vi "CLD 11 Producer consumer events solution.vi"() -> ()   [LabVIEW 2018]
doc: "CLD 11 exercise.\n\nThis VI uses the producer consumer architecture with an event structure. Since there was only one data value (time target) to be used, monitoring changes for the time target control is done with polling instead of the event structure."
uses:
  CLD 11 producer consumer enum.ctl
  CLD 11 CSV file data structure.ctl
  CLD 11 Producer Consumer Data Structure.ctl
  CLD 11 CSV file enum.ctl
panel:
  out "Current Time target":dbl
  out "Elapsed Time (s)":dbl
  out "Step 3":bool
  out "Step 2":bool
  out "Step 1":bool
  out "Time Has Elapsed":bool
  in  "Auto Reset":bool=TRUE
  in  "Reset Button":bool
  in  "Stop VI":bool
  in  "Time Target (s)":dbl
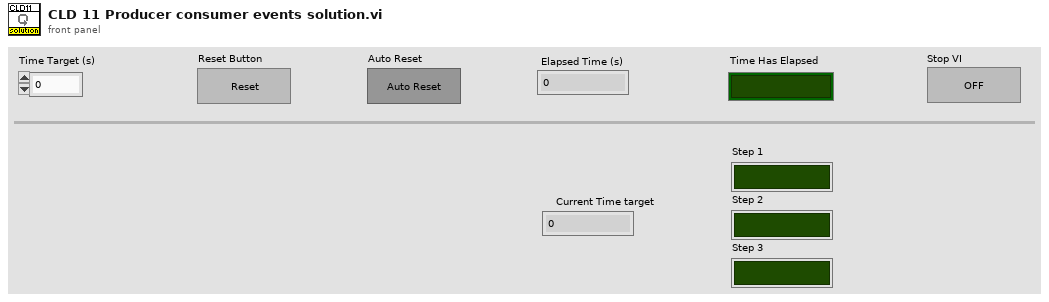
[diagram p1: front panel]
types:
  T1 = typedef "CLD 11 Producer Consumer Data Structure.ctl" = cluster{"CSV File Data Structure":T2, "Time has Elapsed":bool, "Reset":bool, "Autoreset":bool, "Time Target (s)":dbl, "Current State Number":i32}
  T2 = typedef "CLD 11 CSV file data structure.ctl" = cluster{"Dwell Time":i32, "State 1":bool, "State 2":bool, "State 3":bool}
  T3 = typedef "CLD 11 producer consumer enum.ctl" = enum16{"Initialize App", "Read CSV File", "Check Timer", "Run State One", "Run State Two", "Run State Three", "Stop App", "Reset", "Autoreset"}
  T4 = typedef "CLD 11 CSV file enum.ctl" = enum16{"Read CSV", "Write CSV"}
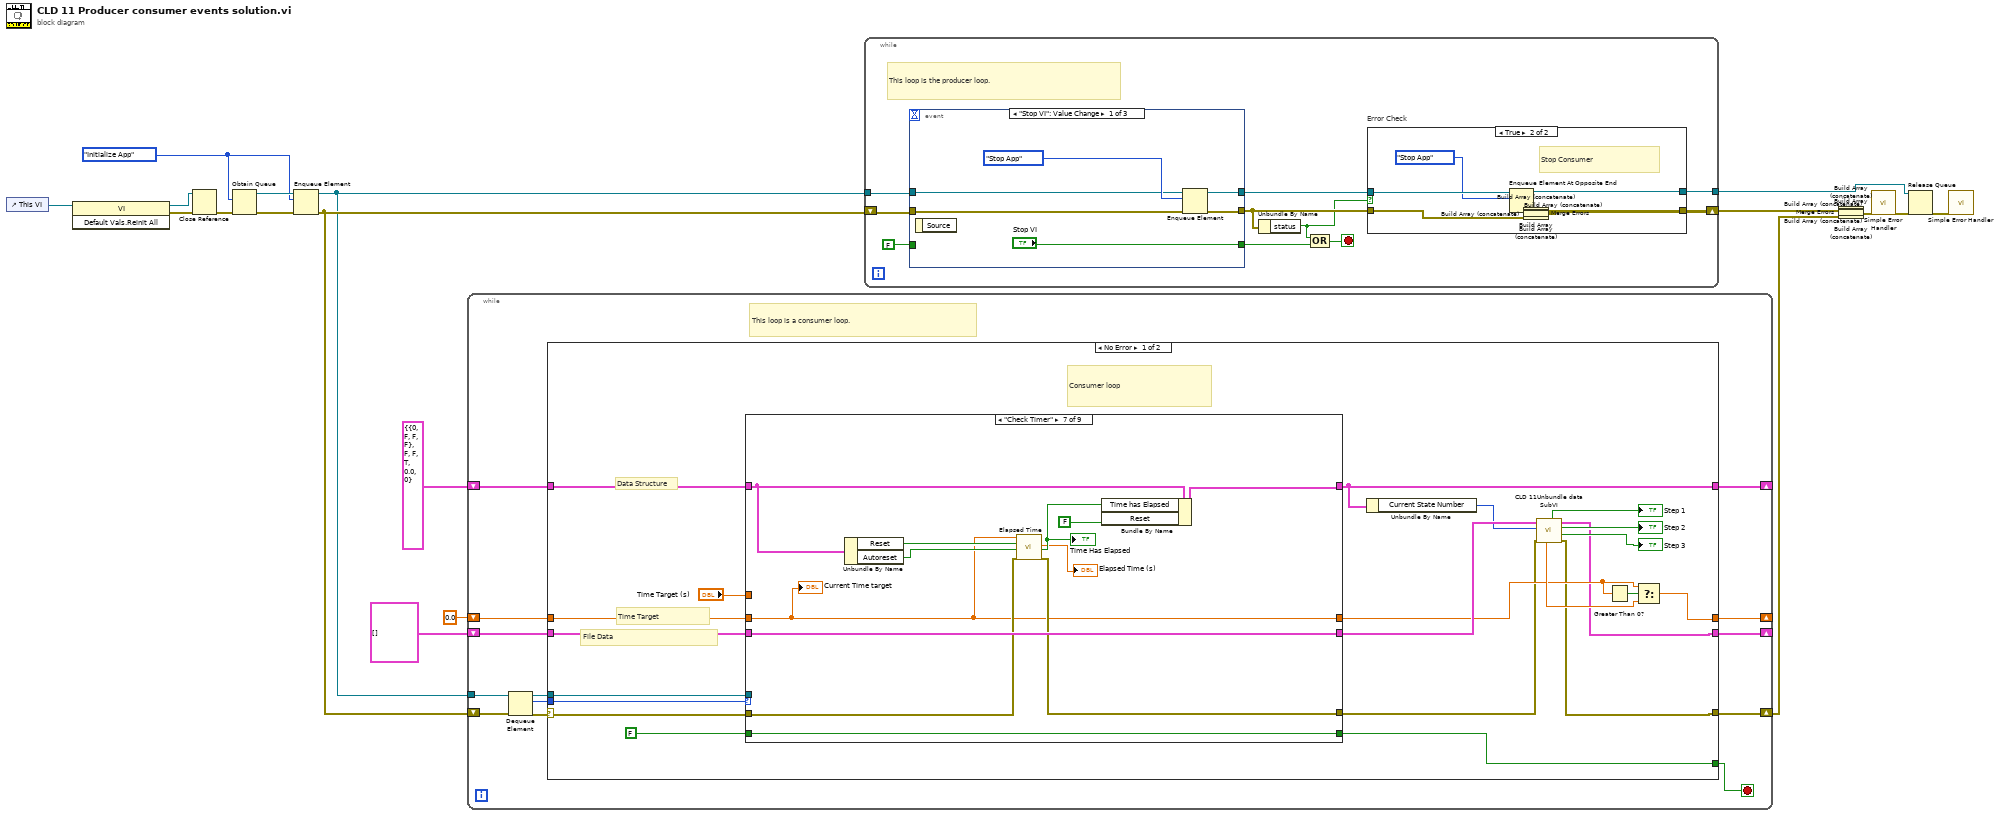
[diagram p0: block diagram]
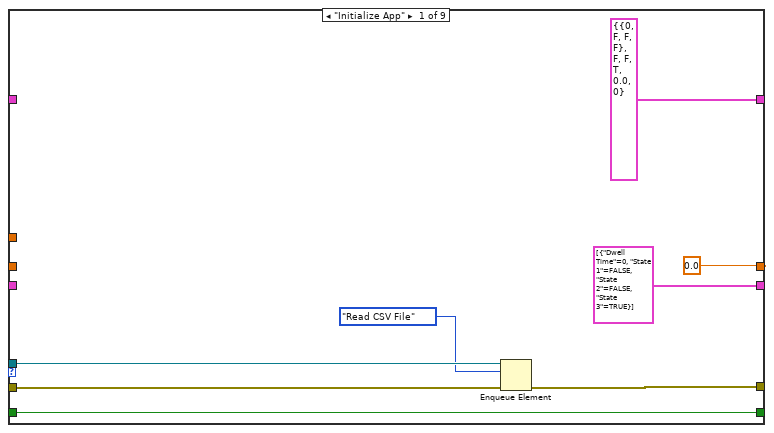
[diagram p2: hidden frame]
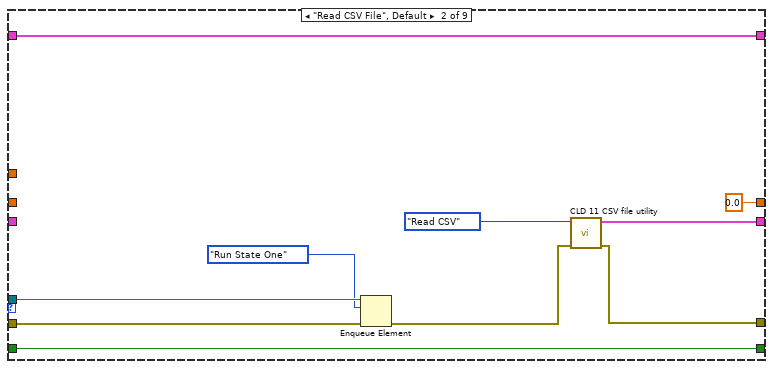
[diagram p3: hidden frame]
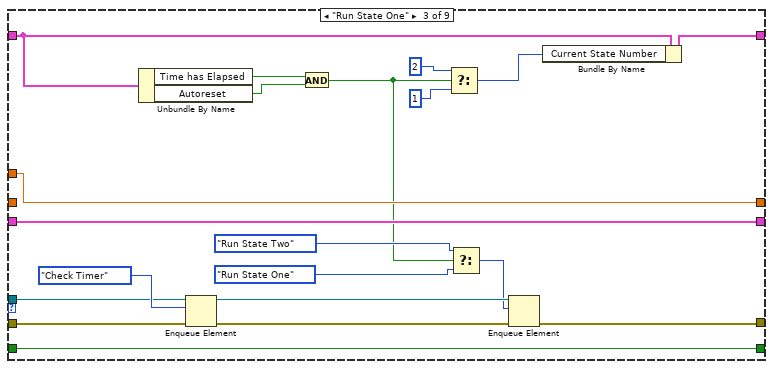
[diagram p4: hidden frame]
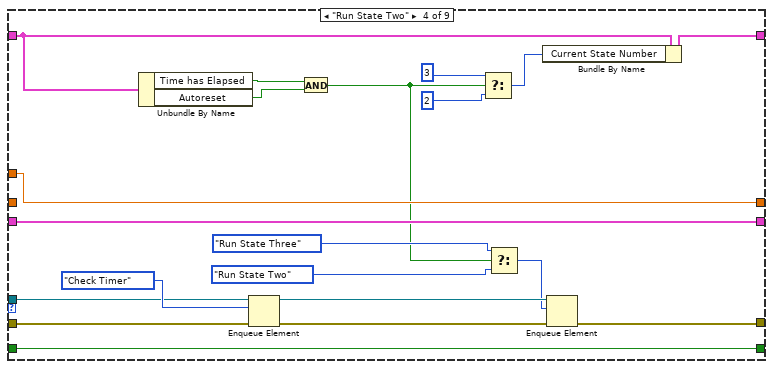
[diagram p5: hidden frame]
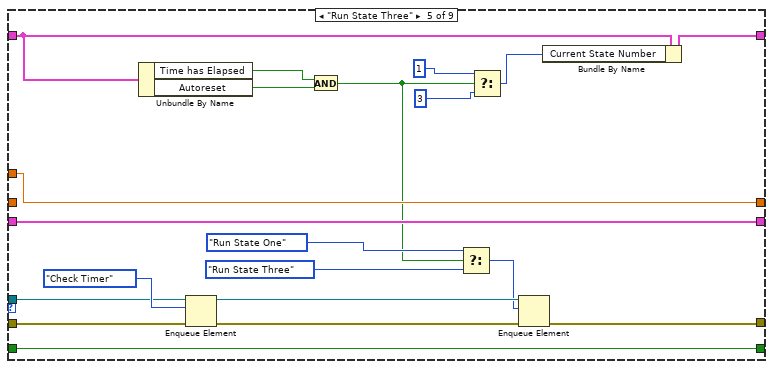
[diagram p6: hidden frame]
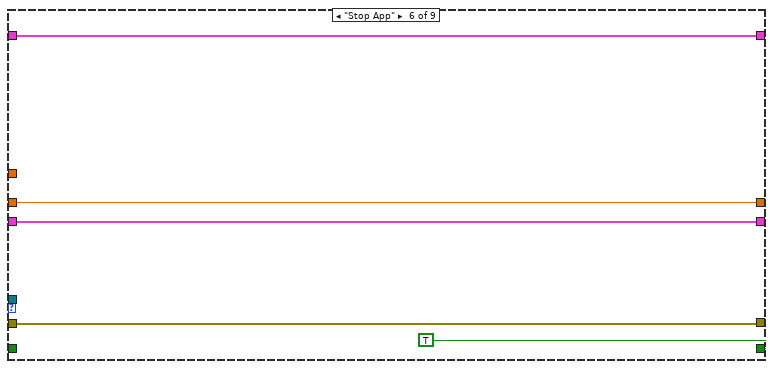
[diagram p7: hidden frame]
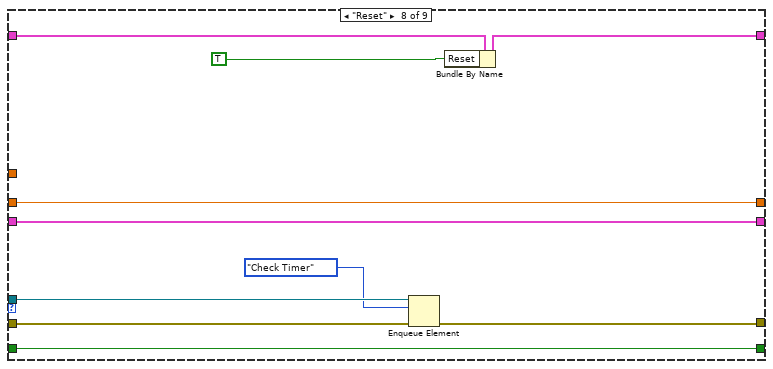
[diagram p8: hidden frame]
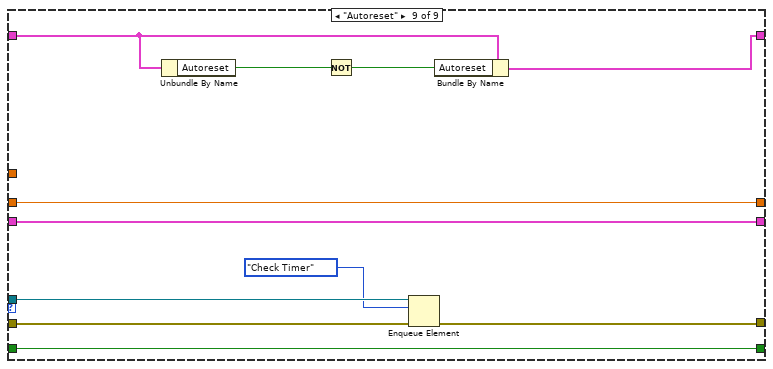
[diagram p9: hidden frame]
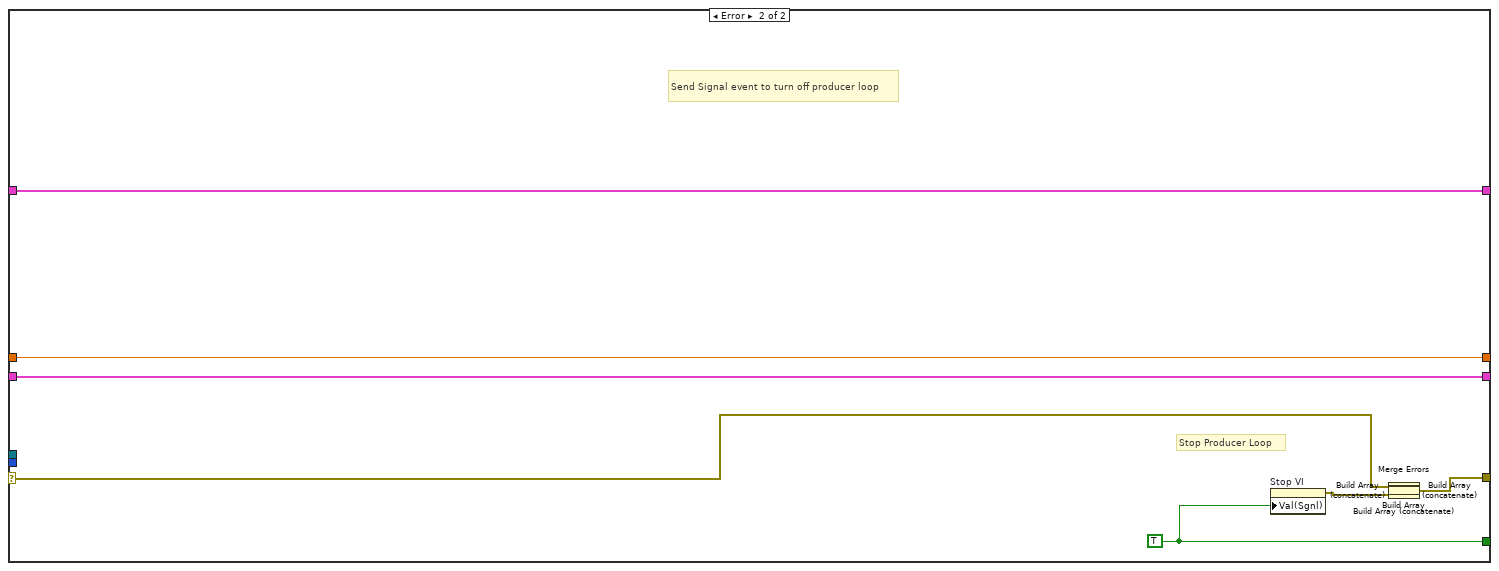
[diagram p10: hidden frame]
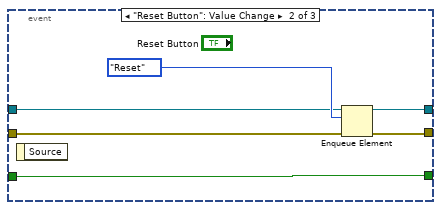
[diagram p12: hidden frame]
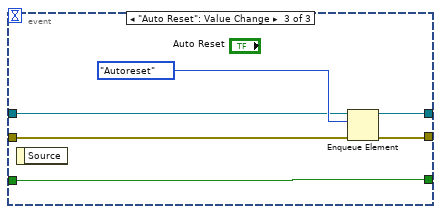
[diagram p13: hidden frame]
diagram:
  w15 = CLD_11_producer_consumer_enum."Initialize App" ("CLD Eighth One Timer Enum")
  n1 = control-ref of="This VI"() -> (w21:refnum<vi>)
  n2 = invoke class="VI" method="Default Vals.Reinit All"(reference=w21) -> (reference out=w19:refnum<vi>, error out=w20:errorcluster)  [unwired: 2 in, 1 out]
  n3 = Close Reference(reference=w19, error in (no error)=w20) -> (error out=w18:errorcluster)
  n4 = Obtain Queue(element data type=w15, error in (no error)=w18) -> (queue out=w22:refnum<queue>, error out=w17:errorcluster)  [unwired: 3 in, 1 out]
  n5 = Enqueue Element(queue=w22, element=w15, error in (no error)=w17) -> (queue out=w7:refnum<queue>, error out=w16:errorcluster)  [unwired: 1 in, 1 out]
  n6 = while {
    tunnel: w7 -> [w36]
    shift-right: [w31] -> w13
    shift-left: w16 -> [w30]
    shift-right: [w29] -> _
    shift-left: T2[] [] ("[Data Out]") -> [w28]
    shift-right: [w27] -> _
    shift-left: 0.0 -> [w26]
    shift-right: [w25] -> _
    shift-left: T1 {"CSV File Data Structure"={"Dwell Time"=0, "State 1"=FALSE, "State 2"=FALSE, "State 3"=FALSE}, "Time has Elapsed"=FALSE, "Reset"=FALSE, "Autoreset"=TRUE, "Time Target (s)"=0.0, "Current State Number"=0} ("Producer Consumer Data Structure") -> [w24]
    stop <- w33 stop-if-true
    # "This loop is a consumer loop."
    n7 = Dequeue Element(queue=w36, error in (no error)=w30) -> (queue out=w32:refnum<queue>, element=w34:T3, error out=w35:errorcluster)  [unwired: 1 in, 1 out]
    n8 = case shown="No Error" w35 {
      selector: w35 -> [w54 w180]
      tunnel: w34 -> [w56 _]
      tunnel: [w58 w182] -> w33
      tunnel: w32 -> [w55 _]
      tunnel: [w39 w181] -> w31
      tunnel: [w37 w184] -> w29
      tunnel: w28 -> [w53 w184]
      tunnel: [w45 w185] -> w27
      tunnel: w26 -> [w52 w185]
      tunnel: [w44 w183] -> w25
      tunnel: w24 -> [w51 w183]
      frame No Error {
        # "File Data"
        # "Time Target"
        # "Data Structure"
        # "Consumer loop"
        n9 = case shown="\"Check Timer\"" w56 {
          tunnel: [w66 w76 w96 w116 w136 TRUE w153 w163 w174] -> w58
          tunnel: FALSE -> [w66 w76 w96 w116 w136 _ w153 w163 w174]
          tunnel: w55 -> [w63 w74 w93 w113 w133 _ _ w158 w171]
          tunnel: w54 -> [w65 w75 w91 w111 w131 w138 w151 w157 w170]
          tunnel: [w64 w69 w89 w109 w129 w138 w150 w156 w169] -> w40
          tunnel: [T2[] [{"Dwell Time"=0, "State 1"=FALSE, "State 2"=FALSE, "State 3"=TRUE}] ("[Data Out]") w72 w95 w115 w135 w141 w152 w162 w173] -> w47
          tunnel: w53 -> [_ _ w95 w115 w135 w141 w152 w162 w173]
          tunnel: [0.0 0.0 ("Dwell Time") w84 w104 w125 w140 w143 w154 w167] -> w46
          tunnel: w52 -> [_ _ _ _ _ w140 w143 w154 w167]
          tunnel: [T1 {"CSV File Data Structure"={"Dwell Time"=0, "State 1"=FALSE, "State 2"=FALSE, "State 3"=FALSE}, "Time has Elapsed"=FALSE, "Reset"=FALSE, "Autoreset"=TRUE, "Time Target (s)"=0.0, "Current State Number"=0} ("Producer Consumer Data Structure") w67 w83 w103 w124 w139 w148 w161 w172] -> w44
          tunnel: w51 -> [_ w67 w88 w108 w128 w139 w147 w160 w166]
          tunnel: "Time Target (s)" -> [_ _ w84 w104 w125 _ _ _ _]
          frame "Initialize App" {
            n10 = Enqueue Element(queue=w63, element=CLD_11_producer_consumer_enum."Read CSV File" ("CLD Eighth One Timer Enum"), error in (no error)=w65) -> (error out=w64:errorcluster)  [unwired: 1 in, 2 out]
          }
          frame "Read CSV File", Default {
            n11 = Enqueue Element(queue=w74, element=CLD_11_producer_consumer_enum."Run State One" ("CLD Eighth One Timer Enum"), error in (no error)=w75) -> (error out=w70:errorcluster)  [unwired: 1 in, 2 out]
            n12 = call "CLD 11 CSV file utility.vi"("Error In"=w70, "CSV File Enum"=CLD_11_CSV_file_enum."Read CSV") -> ("Error Out"=w69:errorcluster, "[Data Out]"=w72:T2[])  [unwired: 8 in]
          }
          frame "Run State One" {
            n13 = Unbundle By Name(w88) -> ("Time has Elapsed"=w78:bool, "Autoreset"=w79:bool)
            n14 = Enqueue Element(queue=w93, element=CLD_11_producer_consumer_enum."Check Timer" ("CLD Eighth One Timer Enum"), error in (no error)=w91) -> (queue out=w92:refnum<queue>, error out=w90:errorcluster)  [unwired: 1 in, 1 out]
            n15 = And(x=w78, y=w79) -> (x .and. y?=w77:bool)
            n16 = Select(t=2 ("Current State Number"), s=w77, f=1 ("Current State Number")) -> (s? t:f=w80:i32)
            n17 = Select(t=CLD_11_producer_consumer_enum."Run State Two" ("CLD Eighth One Timer Enum"), s=w77, f=CLD_11_producer_consumer_enum."Run State One" ("CLD Eighth One Timer Enum")) -> (s? t:f=w85:T3)
            n18 = Enqueue Element(queue=w92, element=w85, error in (no error)=w90) -> (error out=w89:errorcluster)  [unwired: 1 in, 2 out]
            n19 = Bundle By Name(cluster=w88, "Current State Number"=w80) -> (w83:T1)
          }
          frame "Run State Two" {
            n20 = Unbundle By Name(w108) -> ("Time has Elapsed"=w98:bool, "Autoreset"=w99:bool)
            n21 = Enqueue Element(queue=w113, element=CLD_11_producer_consumer_enum."Check Timer" ("CLD Eighth One Timer Enum"), error in (no error)=w111) -> (queue out=w112:refnum<queue>, error out=w110:errorcluster)  [unwired: 1 in, 1 out]
            n22 = And(x=w98, y=w99) -> (x .and. y?=w97:bool)
            n23 = Select(t=3 ("Current State Number"), s=w97, f=2 ("Current State Number")) -> (s? t:f=w100:i32)
            n24 = Select(t=CLD_11_producer_consumer_enum."Run State Three" ("CLD Eighth One Timer Enum"), s=w97, f=CLD_11_producer_consumer_enum."Run State Two" ("CLD Eighth One Timer Enum")) -> (s? t:f=w105:T3)
            n25 = Bundle By Name(cluster=w108, "Current State Number"=w100) -> (w103:T1)
            n26 = Enqueue Element(queue=w112, element=w105, error in (no error)=w110) -> (error out=w109:errorcluster)  [unwired: 1 in, 2 out]
          }
          frame "Run State Three" {
            n27 = Unbundle By Name(w128) -> ("Time has Elapsed"=w118:bool, "Autoreset"=w119:bool)
            n28 = Enqueue Element(queue=w133, element=CLD_11_producer_consumer_enum."Check Timer" ("CLD Eighth One Timer Enum"), error in (no error)=w131) -> (queue out=w132:refnum<queue>, error out=w130:errorcluster)  [unwired: 1 in, 1 out]
            n29 = And(x=w118, y=w119) -> (x .and. y?=w117:bool)
            n30 = Select(t=CLD_11_producer_consumer_enum."Run State One" ("CLD Eighth One Timer Enum"), s=w117, f=CLD_11_producer_consumer_enum."Run State Three" ("CLD Eighth One Timer Enum")) -> (s? t:f=w126:T3)
            n31 = Select(t=1 ("Current State Number"), s=w117, f=3 ("Current State Number")) -> (s? t:f=w121:i32)
            n32 = Enqueue Element(queue=w132, element=w126, error in (no error)=w130) -> (error out=w129:errorcluster)  [unwired: 1 in, 2 out]
            n33 = Bundle By Name(cluster=w128, "Current State Number"=w121) -> (w124:T1)
          }
          frame "Stop App" {
          }
          frame "Check Timer" {
            n34 = Unbundle By Name(w147) -> ("Reset"=w146:bool, "Autoreset"=w145:bool)
            n35 = call "Elapsed Time"("Time Target (s)"=w143, "Reset"=w146, "Auto Reset"=w145, "error in (no error)"=w151) -> ("Elapsed Time (s)"=→"Elapsed Time (s)":dbl, "Time has Elapsed"=w149:bool, "error out"=w150:errorcluster)  [unwired: 8 in, 5 out]
            "Time Has Elapsed" <- w149
            n36 = Bundle By Name(cluster=w147, "Time has Elapsed"=w149, "Reset"=FALSE) -> (w148:T1)
            "Current Time target" <- w143
          }
          frame "Reset" {
            n37 = Enqueue Element(queue=w158, element=CLD_11_producer_consumer_enum."Check Timer", error in (no error)=w157) -> (error out=w156:errorcluster)  [unwired: 1 in, 2 out]
            n38 = Bundle By Name(cluster=w160, "Reset"=TRUE) -> (w161:T1)
          }
          frame "Autoreset" {
            n39 = Unbundle By Name(w166) -> ("Autoreset"=w165:bool)
            n40 = Not(x=w165) -> (.not. x?=w164:bool)
            n41 = Enqueue Element(queue=w171, element=CLD_11_producer_consumer_enum."Check Timer", error in (no error)=w170) -> (error out=w169:errorcluster)  [unwired: 1 in, 2 out]
            n42 = Bundle By Name(cluster=w166, "Autoreset"=w164) -> (w172:T1)
          }
        }
        n43 = Unbundle By Name(w44) -> ("Current State Number"=w43:i32)
        n44 = call "CLD 11Unbundle data SubVI.vi"("error in (no error)"=w40, "Current State Number"=w43, "[Data In]"=w47) -> ("error out"=w39:errorcluster, "State 3"=→"Step 3":bool, "State 2"=→"Step 2":bool, "[Data Out]"=w37:T2[], "State 1"=→"Step 1":bool, "Dwell Time"=w49:dbl)  [unwired: 2 in, 1 out]
        n45 = Greater Than 0?(x=w46) -> (x > 0?=w48:bool)
        n46 = Select(t=w46, s=w48, f=w49) -> (s? t:f=w45:dbl)
      }
      frame Error {
        w182 = TRUE
        # "Stop Producer Loop"
        # "Send Signal event to turn off producer loop"
        n47 = property on="Stop VI" class="Bool (strict)"("Val(Sgnl)"=w182) -> (error out=w179:errorcluster)  [unwired: 2 in, 1 out]
        n48 = Build Array(w180, w179) -> (w178:errorcluster[])
        n49 = Build Array (concatenate)(w178) -> (w177:errorcluster[])
        n50 = Build Array (concatenate)(w177) -> (w176:errorcluster[])
        n51 = Build Array (concatenate)(w176) -> (w175:errorcluster[])
        n52 = Merge Errors(w175) -> (w181:errorcluster)
      }
    }
  }
  n53 = while {
    tunnel: w7 -> [w195]
    tunnel: [w186] -> w6
    shift-right: [w191] -> w23
    shift-left: w16 -> [w194]
    stop <- w187 stop-if-true
    # "This loop is the producer loop."
    n54 = event shown="[0] \"Stop VI\": Value Change" {
      selector: _ -> [_ _ _]
      dyn-events: _ -> [_ _ _]
      timeout: _ -> [_ _ _]
      tunnel: w195 -> [w210 w217 w223]
      tunnel: w194 -> [w213 w220 w226]
      tunnel: [w212 w219 w225] -> w189
      tunnel: ["Stop VI" w216 w222] -> w193
      tunnel: FALSE ("stop VI") -> [_ w216 w222]
      tunnel: [w209 w215 w221] -> w190
      event "Stop VI": Value Change {
        n55 = event-data() -> ()  [unwired: 1 in, 1 out]
        n56 = Enqueue Element(queue=w210, element=CLD_11_producer_consumer_enum."Stop App" ("CLD Eighth One Timer Enum"), error in (no error)=w213) -> (queue out=w209:refnum<queue>, error out=w212:errorcluster)  [unwired: 1 in, 1 out]
      }
      event "Reset Button": Value Change {
        n57 = event-data() -> ()  [unwired: 1 in, 1 out]
        n58 = Enqueue Element(queue=w217, element=CLD_11_producer_consumer_enum."Reset" ("CLD Eighth One Timer Enum"), error in (no error)=w220) -> (queue out=w215:refnum<queue>, error out=w219:errorcluster)  [unwired: 1 in, 1 out]
      }
      event "Auto Reset": Value Change {
        n59 = event-data() -> ()  [unwired: 1 in, 1 out]
        n60 = Enqueue Element(queue=w223, element=CLD_11_producer_consumer_enum."Autoreset" ("CLD Eighth One Timer Enum"), error in (no error)=w226) -> (queue out=w221:refnum<queue>, error out=w225:errorcluster)  [unwired: 1 in, 1 out]
      }
    }
    n61 = Unbundle By Name(w189) -> ("status"=w188:bool)
    n62 = Compound Arithmetic op=OR(w188, w193) -> (w187:bool)
    n63 = case "Error Check" shown="True" w188 {
      tunnel: w189 -> [w197 w204]
      tunnel: [w197 w205] -> w191
      tunnel: w190 -> [w196 w207]
      tunnel: [w196 w203] -> w186
      frame False {
      }
      frame True {
        # "Stop Consumer"
        n64 = Enqueue Element At Opposite End(queue=w207, element=CLD_11_producer_consumer_enum."Stop App" ("CLD Eighth One Timer Enum")) -> (queue out=w203:refnum<queue>, error out=w208:errorcluster)  [unwired: 2 in, 1 out]
        n65 = Build Array(w208, w204) -> (w202:errorcluster[])
        n66 = Build Array (concatenate)(w202) -> (w201:errorcluster[])
        n67 = Build Array (concatenate)(w201) -> (w200:errorcluster[])
        n68 = Build Array (concatenate)(w200) -> (w199:errorcluster[])
        n69 = Build Array (concatenate)(w199) -> (w198:errorcluster[])
        n70 = Merge Errors(w198) -> (w205:errorcluster)
      }
    }
  }
  n71 = Build Array(w23, w13) -> (w5:errorcluster[])
  n72 = Build Array (concatenate)(w5) -> (w4:errorcluster[])
  n73 = Build Array (concatenate)(w4) -> (w3:errorcluster[])
  n74 = Build Array (concatenate)(w3) -> (w2:errorcluster[])
  n75 = Build Array (concatenate)(w2) -> (w1:errorcluster[])
  n76 = Merge Errors(w1) -> (w14:errorcluster)
  n77 = call <vilib>:"Simple Error Handler.vi"("error in (no error)"=w14) -> ("error out"=w12:errorcluster)  [unwired: 4 in, 4 out]
  n78 = Release Queue(queue=w6, error in (no error)=w12) -> (error out=w8:errorcluster)  [unwired: 1 in, 2 out]
  n79 = call <vilib>:"Simple Error Handler.vi"("error in (no error)"=w8) -> ()  [unwired: 4 in, 5 out]
